vi "Temperature device cluster to String.vi"(11 "Temperature Device Settings":T1) -> (3 "Data to send":string="EXCT:TYPE:Unipolar:MAG:10.00:EXCT:NICK:MB1.T1:LOOP:AUX:None:PSET:1.0:HTR:None:ISET:1.0:HAUT:Manual:HSET:0.0:PIDT:Manual:DSET:1.0:TSET:0K:LVL:MB1.T1:LOOP:MAN:HVER:0:FVER:20.6:SERL:102750119:MAN:CAL:OFFS:0.0000:COLD:1.0000:INT:Linear:SCAL:1.0000:FILE:RP5.DAT:HOTL:1023.1500:CAL:TYPE:PTC:SIG:VOLT:1405.9mV:CURR:10µA:TEMP:1023.15K:POWR:14.059µW:RES:140590?:SLOP:137.409?/K:FLOW:NOT_FOUND:SIG:TEMP\n")   [LabVIEW 2015, in "Mercury iXX.lvlib" / "Temperature.lvlib"]
uses:
  Temperature.lvlib
  Controls/Temperature Device (Set).ctl
  Controls/Temperature Sensor Type.ctl
  Controls/Excitation Cluster.ctl
  Controls/Excitation Type.ctl
  Controls/Calibration Cluster.ctl
  Controls/Calibration Interpolation.ctl
  Controls/Loop Cluster.ctl
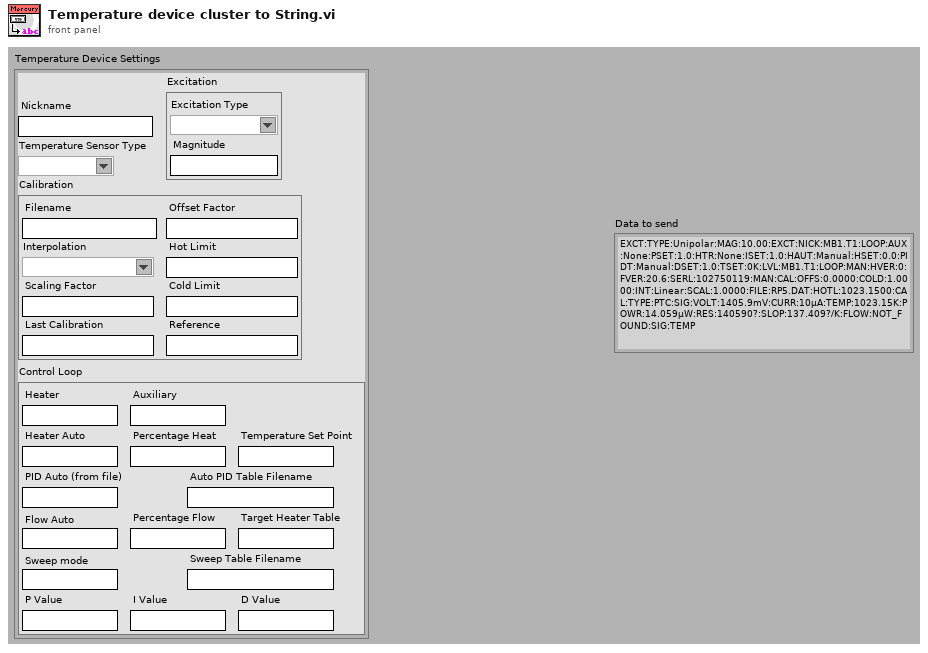
[diagram p1: front panel]
types:
  T1 = typedef "Mercury iXX.lvlib/Temperature.lvlib/Temperature Device (Set).ctl" = cluster{"Nickname":string, "Temperature Sensor Type":T2, "Excitation":T3, "Calibration":T5, "Control Loop":T7}
  T2 = typedef "Mercury iXX.lvlib/Temperature.lvlib/Temperature Sensor Type.ctl" = string
  T3 = typedef "Mercury iXX.lvlib/Temperature.lvlib/Excitation Cluster.ctl" = cluster{"Excitation Type":T4, "Magnitude":string}
  T4 = typedef "Mercury iXX.lvlib/Temperature.lvlib/Excitation Type.ctl" = string
  T5 = typedef "Mercury iXX.lvlib/Temperature.lvlib/Calibration Cluster.ctl" = cluster{"Filename":string, "Interpolation":T6, "Scaling Factor":string, "Offset Factor":string, "Hot Limit":string, "Cold Limit":string, "Last Calibration":string, "Reference":string}
  T6 = typedef "Mercury iXX.lvlib/Temperature.lvlib/Calibration Interpolation.ctl" = string
  T7 = typedef "Mercury iXX.lvlib/Temperature.lvlib/Loop Cluster.ctl" = cluster{"Heater":string, "Auxiliary":string, "Heater Auto":string, "Percentage Heat":string, "Temperature Set Point":string, "PID Auto (from file)":string, "P Value":string, "I Value":string, "D Value":string, "Auto PID Table Filename":string, "Flow Auto":string, "Target Heater Table":string, "Sweep mode":string, "Sweep Table Filename":string, "Percentage Flow":string}
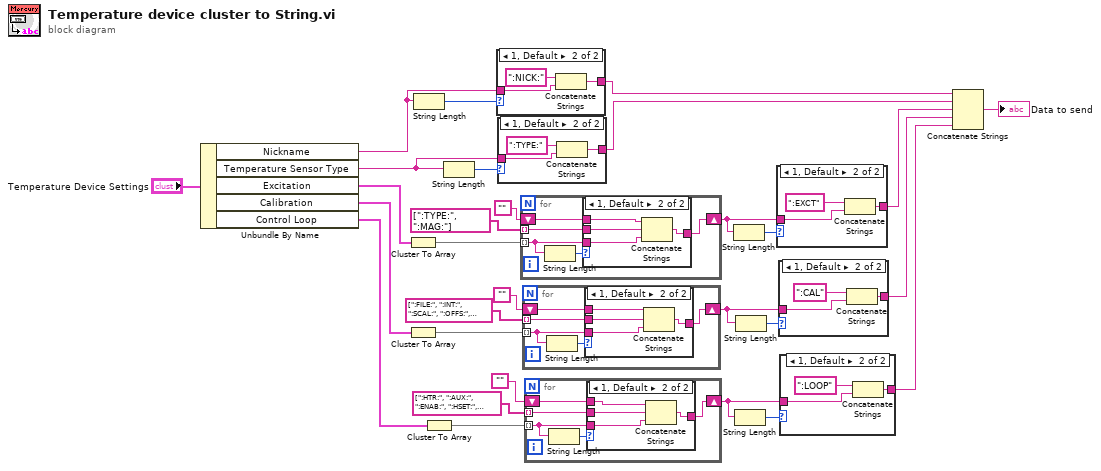
[diagram p0: block diagram]
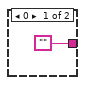
[diagram p2: hidden frame]
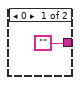
[diagram p3: hidden frame]
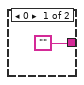
[diagram p4: hidden frame]
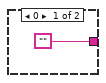
[diagram p8: hidden frame]
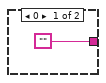
[diagram p9: hidden frame]
diagram:
  n1 = Unbundle By Name("Temperature Device Settings") -> ("Nickname"=w24:string, "Temperature Sensor Type"=w22:T2, "Excitation"=w28:T3, "Calibration"=w27:T5, "Control Loop"=w26:T7)
  n2 = Cluster To Array(cluster=w28) -> (array=w18:T4[])
  n3 = Cluster To Array(cluster=w27) -> (array=w14:T6[])
  n4 = String Length(string=w24) -> (length=w25:i32)
  n5 = Cluster To Array(cluster=w26) -> (array=w12:string[])
  n6 = String Length(string=w22) -> (length=w23:i32)
  n7 = case shown="1, Default" w25 {
    tunnel: w24 -> [_ w32]
    tunnel: ["" w33] -> w21
    frame 0 {
    }
    frame 1, Default {
      n8 = Concatenate Strings(":NICK:" ("string"), w32) -> (w33:string)
    }
  }
  n9 = case shown="1, Default" w23 {
    tunnel: w22 -> [_ w36]
    tunnel: ["" w37] -> w20
    frame 0 {
    }
    frame 1, Default {
      n10 = Concatenate Strings(":TYPE:" ("string"), w36) -> (w37:string)
    }
  }
  n11 = for {
    tunnel: w18 -> [w41] mode=indexing
    tunnel: string[] [":TYPE:", ":MAG:"] ("Excitation") -> [w40] mode=indexing
    shift-right: [w39] -> w3
    shift-left: "" -> [w38]
    n12 = String Length(string=w41) -> (length=w42:i32)
    n13 = case shown="1, Default" w42 {
      tunnel: w41 -> [_ w46]
      tunnel: [w43 w47] -> w39
      tunnel: w40 -> [_ w45]
      tunnel: w38 -> [w43 w44]
      frame 0 {
      }
      frame 1, Default {
        n14 = Concatenate Strings(w44, w45, w46) -> (w47:string)
      }
    }
  }
  n15 = for {
    tunnel: w14 -> [w51] mode=indexing
    tunnel: string[] [":FILE:", ":INT:", ":SCAL:", ":OFFS:", ":HOTL:", ":COLDL:"] ("Excitation") -> [w50] mode=indexing
    shift-right: [w49] -> w6
    shift-left: "" -> [w48]
    n16 = String Length(string=w51) -> (length=w52:i32)
    n17 = case shown="1, Default" w52 {
      tunnel: w51 -> [_ w56]
      tunnel: [w53 w57] -> w49
      tunnel: w50 -> [_ w55]
      tunnel: w48 -> [w53 w54]
      frame 0 {
      }
      frame 1, Default {
        n18 = Concatenate Strings(w54, w55, w56) -> (w57:string)
      }
    }
  }
  n19 = for {
    tunnel: w12 -> [w61] mode=indexing
    tunnel: string[] [":HTR:", ":AUX:", ":ENAB:", ":HSET:", ":TSET:", ":PIDT:", ":P:", ":I:", ":D:", ":PIDF:", ":FAUT:", ":THTF:", ":SWMD:", ":SWFL:", ":FSET:"] ("Excitation") -> [w60] mode=indexing
    shift-right: [w59] -> w5
    shift-left: "" -> [w58]
    n20 = String Length(string=w61) -> (length=w62:i32)
    n21 = case shown="1, Default" w62 {
      tunnel: w61 -> [_ w66]
      tunnel: [w63 w67] -> w59
      tunnel: w60 -> [_ w65]
      tunnel: w58 -> [w63 w64]
      frame 0 {
      }
      frame 1, Default {
        n22 = Concatenate Strings(w64, w65, w66) -> (w67:string)
      }
    }
  }
  n23 = String Length(string=w3) -> (length=w4:i32)
  n24 = String Length(string=w5) -> (length=w1:i32)
  n25 = String Length(string=w6) -> (length=w2:i32)
  n26 = case shown="1, Default" w4 {
    tunnel: ["" w71] -> w16
    tunnel: w3 -> [_ w70]
    frame 0 {
    }
    frame 1, Default {
      n27 = Concatenate Strings(":EXCT" ("string"), w70) -> (w71:string)
    }
  }
  n28 = case shown="1, Default" w2 {
    tunnel: ["" w75] -> w11
    tunnel: w6 -> [_ w74]
    frame 0 {
    }
    frame 1, Default {
      n29 = Concatenate Strings(":CAL" ("string"), w74) -> (w75:string)
    }
  }
  n30 = case shown="1, Default" w1 {
    tunnel: ["" w79] -> w10
    tunnel: w5 -> [_ w78]
    frame 0 {
    }
    frame 1, Default {
      n31 = Concatenate Strings(":LOOP" ("string"), w78) -> (w79:string)
    }
  }
  n32 = Concatenate Strings(w21, w20, w16, w11, w10) -> (→"Data to send":string)
